vi "Finish.vi"   [LabVIEW 2015]
doc: "This VI is called just before exiting. It is expected to close I/O refnum, save collected data, etc."
uses:
  <vilib>/Rock Robotics/WPI/Utilities/WPI_GetSetVariantRefNum.vi
types:
  T1 = typedef "WPI_AccelerometerDevRef.ctl" = cluster{"DevStatus":errorcluster, "Scaling":T2, "Analog Channels":T3, "I2C Bus":T5, "SPI Bus":T6, "Accel Range":T7, "ADXL Axes":T8, "Handle":i32, "Device Address":u8, "Accel Type":enum16{"Analog", "ADXL345 I2C", "ADXL345 SPI", "Internal", "ADXL362 SPI"}}
  T2 = typedef "WPI_AccelerometerScaling.ctl" = cluster{"Gain (VoltsPerG)":dbl, "Center Voltage":dbl}
  T3 = typedef "WPI_AccelerometerAnalogChannels.ctl" = cluster{"X-Axis":T4, "Y-Axis":T4, "Z-Axis":T4}
  T4 = typedef "FPGA_AIChannel.ctl" = enum8{"AI 0", "AI 1", "AI 2", "AI 3", "AI MXP 0", "AI MXP 1", "AI MXP 2", "AI MXP 3", "Invalid"}
  T5 = typedef "i2c_bus.ctl" = enum16{"I2C On-Board", "I2C MXP", "Invalid"}
  T6 = typedef "spi_bus.ctl" = enum16{"SPI On-Board, CS0", "SPI On-Board, CS1", "SPI On-Board, CS2", "SPI On-Board, CS3", "SPI MXP", "Invalid"}
  T7 = typedef "ADXL345 Range.ctl" = u8
  T8 = typedef "WPI_AccelerometerADXL345 Axes.ctl" = cluster{"X-Axis":bool, "Y-Axis":bool, "Z-Axis":bool}
  T9 = typedef "WPI_DigitalInputDevRef.ctl" = cluster{"DevStatus":errorcluster, "DIO Channel":T10}
  T10 = typedef "FPGA_DIOChannel.ctl" = enum8{"DIO 0", "DIO 1", "DIO 2", "DIO 3", "DIO 4", "DIO 5", "DIO 6", "DIO 7", "DIO 8", "DIO 9", "DIO MXP 0", "DIO MXP 1", "DIO MXP 2", "DIO MXP 3", "DIO MXP 4", "DIO MXP 5", "DIO MXP 6", "DIO MXP 7", "DIO MXP 8", "DIO MXP 9", "DIO MXP 10", "DIO MXP 11", "DIO MXP 12", "DIO MXP 13", "DIO MXP 14", "DIO MXP 15", "Invalid"}
  T11 = typedef "WPI_GyroDevRef.ctl" = cluster{"DevStatus":errorcluster, "Analog Channel":T4, "Offset":dbl, "Gain (VoltsPerDegree/Second)":dbl, "Gyro Type":enum16{"Analog", "XRS450"}, "Handle":i32, "SPI Bus":T6, "Device Found":bool, "Sample Rate":dbl, "Calibrate On Open":bool}
  T12 = typedef "WPI_RelayDevRef.ctl" = cluster{"DevStatus":errorcluster, "Relay Channel":T13, "Relay Direction":T14}
  T13 = typedef "FPGA_DIORelayChannel.ctl" = enum8{"Relay 0", "Relay 1", "Relay 2", "Relay 3", "Invalid"}
  T14 = typedef "WPI_RelayDirection.ctl" = enum16{"Both directions", "Forward only", "Reverse only"}
  T15 = typedef "WPI_SolenoidDevRef.ctl" = cluster{"DevStatus":errorcluster, "Pneumatics Control Module":u8, "Forward Solenoid Channel":T16, "Reverse Solenoid Channel":T16}
  T16 = typedef "WPI_SolenoidChannel.ctl" = enum8{"Solenoid 0", "Solenoid 1", "Solenoid 2", "Solenoid 3", "Solenoid 4", "Solenoid 5", "Solenoid 6", "Solenoid 7", "Invalid"}
  T17 = typedef "WPI_EncoderDevRef.ctl" = cluster{"DevStatus":errorcluster, "EncoderIndex":T18, "CounterIndex":T19, "DistancePerCount":dbl, "Decoding Type":T20}
  T18 = typedef "FPGA_EncoderIdx.ctl" = enum8{"Enc 0", "Enc 1", "Enc 2", "Enc 3", "Enc 4", "Enc 5", "Enc 6", "Enc 7", "Invalid"}
  T19 = typedef "FPGA_CounterCtrSystemIndex.ctl" = enum8{"Ctr 0", "Ctr 1", "Ctr 2", "Ctr 3", "Ctr 4", "Ctr 5", "Ctr 6", "Ctr 7", "Invalid"}
  T20 = typedef "WPI_EncoderType.ctl" = enum16{"1x", "2x", "4x"}
  T21 = typedef "WPI_PotentiometerDevRef.ctl" = cluster{"DevStatus":errorcluster, "Analog Channel":T4, "Invert Output":bool}
  T22 = typedef "WPI_ServoDeviceRef.ctl" = cluster{"DeviceStatus":errorcluster, "PWM Channel":T23, "DeadBand":T24}
  T23 = typedef "FPGA_DIOPWMChannel.ctl" = enum8{"PWM 0", "PWM 1", "PWM 2", "PWM 3", "PWM 4", "PWM 5", "PWM 6", "PWM 7", "PWM 8", "PWM 9", "PWM MXP 0", "PWM MXP 1", "PWM MXP 2", "PWM MXP 3", "PWM MXP 4", "PWM MXP 5", "PWM MXP 6", "PWM MXP 7", "PWM MXP 8", "PWM MXP 9", "Invalid"}
  T24 = typedef "WPI_PWMDeadband.ctl" = cluster{"Name":string, "maxPositivePwm":i32, "minPositivePwm":i32, "centerPwm":i32, "maxNegativePwm":i32, "minNegativePwm":i32, "angularRange":u16}
  T25 = typedef "WPI_JoystickDevRef.ctl" = cluster{"Device":T26}
  T26 = typedef "WPI_JoystickDeviceEnum.ctl" = enum16{"USB 0", "USB 1", "USB 2", "USB 3", "USB 4", "USB 5"}
  T27 = typedef "WPI_MotorControlDeviceRef.ctl" = cluster{"DeviceStatus":errorcluster, "Type":T28, "PWM":cluster{"PWM Channel":T23, "DeadBand":T24}, "CAN":cluster{"Device Number":u8, "Control Mode":T29, "Semaphore":T30, "Max Vout":dbl, "TalonSRX Control Mode":T31}, "Invert":bool}
  T28 = typedef "WPI_MotorControlType.ctl" = enum16{"PWM", "CAN", "CANTalonSRX"}
  T29 = typedef "WPI_CANJaguar_ControlMode.ctl" = enum8{"Percent VBus", "Current", "Speed", "Position", "Voltage"}
  T30 = typedef "Semaphore RefNum" = refnum<k1>
  T31 = typedef "WPI_CANTalonSRX_APIControlMode.ctl" = enum8{"Percent VBus", "Speed", "Position", "Slave", "Unchanged / Invalid", "Voltage Compensation", "Current", "Motion Profile"}
  T32 = typedef "WPI_RobotDriveDevRef.ctl" = cluster{"DevStatus":errorcluster, "Motors[]":T27[], "Square Inputs":bool, "Max Output":dbl}
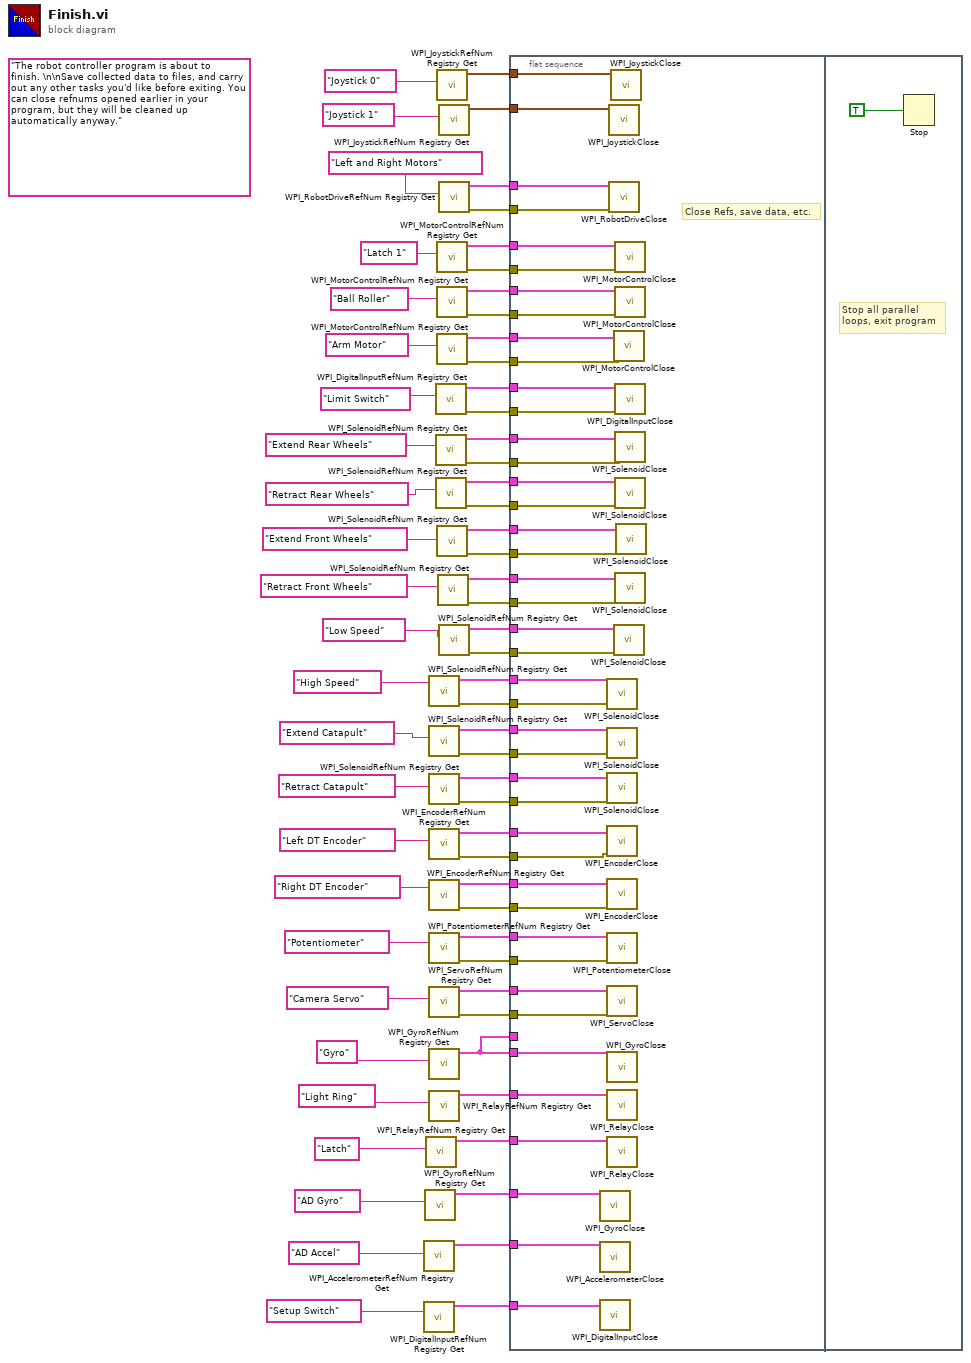
[diagram p0: block diagram]
diagram:
  (unwired) "The robot controller program is about to finish. \n\nSave collected data to files, and carry out any other tasks you'd like before exiting. You can close refnums opened earlier in your program, but they will be cleaned up automatically anyway."
  n1 = call <vilib>:"WPI_AccelerometerRefNum Registry Get.vi"("refnum name"="AD Accel") -> ("AccelerometerDevRef"=w5:T1)  [unwired: 9 in, 1 out]
  n2 = call <vilib>:"WPI_DigitalInputRefNum Registry Get.vi"("refnum name"="Setup Switch") -> ("DigitalInputDevRef"=w2:T9)  [unwired: 9 in, 1 out]
  n3 = call <vilib>:"WPI_GyroRefNum Registry Get.vi"("refnum name"="AD Gyro") -> ("GyroDevRef"=w6:T11)  [unwired: 9 in, 1 out]
  n4 = call <vilib>:"WPI_RelayRefNum Registry Get.vi"("refnum name"="Latch") -> ("RelayDevRef"=w8:T12)  [unwired: 9 in, 1 out]
  n5 = call <vilib>:"WPI_SolenoidRefNum Registry Get.vi"("refnum name"="High Speed") -> ("error out"=w29:errorcluster, "SolenoidDevRef"=w30:T15)  [unwired: 9 in]
  n6 = call <vilib>:"WPI_SolenoidRefNum Registry Get.vi"("refnum name"="Extend Catapult") -> ("error out"=w27:errorcluster, "SolenoidDevRef"=w28:T15)  [unwired: 9 in]
  n7 = call <vilib>:"WPI_SolenoidRefNum Registry Get.vi"("refnum name"="Retract Catapult") -> ("error out"=w25:errorcluster, "SolenoidDevRef"=w26:T15)  [unwired: 9 in]
  n8 = call <vilib>:"WPI_EncoderRefNum Registry Get.vi"("refnum name"="Left DT Encoder") -> ("error out"=w23:errorcluster, "EncoderDevRef"=w24:T17)  [unwired: 9 in]
  n9 = call <vilib>:"WPI_EncoderRefNum Registry Get.vi"("refnum name"="Right DT Encoder") -> ("error out"=w21:errorcluster, "EncoderDevRef"=w22:T17)  [unwired: 9 in]
  n10 = call <vilib>:"WPI_PotentiometerRefNum Registry Get.vi"("refnum name"="Potentiometer") -> ("error out"=w17:errorcluster, "PotDevRef"=w18:T21)  [unwired: 9 in]
  n11 = call <vilib>:"WPI_ServoRefNum Registry Get.vi"("refnum name"="Camera Servo") -> ("error out"=w14:errorcluster, "ServoDeviceRef"=w15:T22)  [unwired: 9 in]
  n12 = call <vilib>:"WPI_GyroRefNum Registry Get.vi"("refnum name"="Gyro") -> ("GyroDevRef"=w11:T11)  [unwired: 9 in, 1 out]
  n13 = call <vilib>:"WPI_RelayRefNum Registry Get.vi"("refnum name"="Light Ring") -> ("RelayDevRef"=w7:T12)  [unwired: 9 in, 1 out]
  n14 = call <vilib>:"WPI_DigitalInputRefNum Registry Get.vi"("refnum name"="Limit Switch") -> ("error out"=w49:errorcluster, "DigitalInputDevRef"=w57:T9)  [unwired: 9 in]
  n15 = call <vilib>:"WPI_SolenoidRefNum Registry Get.vi"("refnum name"="Extend Rear Wheels") -> ("error out"=w52:errorcluster, "SolenoidDevRef"=w53:T15)  [unwired: 9 in]
  n16 = call <vilib>:"WPI_SolenoidRefNum Registry Get.vi"("refnum name"="Retract Rear Wheels") -> ("error out"=w50:errorcluster, "SolenoidDevRef"=w51:T15)  [unwired: 9 in]
  n17 = call <vilib>:"WPI_JoystickRefNum Registry Get.vi"("refnum name"="Joystick 0") -> ("JoystickDevRef"=w58:T25)  [unwired: 1 in, 9 out]
  n18 = call <vilib>:"WPI_MotorControlRefNum Registry Get.vi"("refnum name"="Latch 1") -> ("error out"=w46:errorcluster, "MotorControlDevRef"=w63:T27)  [unwired: 9 in]
  n19 = call <vilib>:"WPI_MotorControlRefNum Registry Get.vi"("refnum name"="Ball Roller") -> ("error out"=w47:errorcluster, "MotorControlDevRef"=w61:T27)  [unwired: 9 in]
  n20 = call <vilib>:"WPI_MotorControlRefNum Registry Get.vi"("refnum name"="Arm Motor") -> ("error out"=w48:errorcluster, "MotorControlDevRef"=w55:T27)  [unwired: 9 in]
  n21 = call <vilib>:"WPI_SolenoidRefNum Registry Get.vi"("refnum name"="Extend Front Wheels") -> ("error out"=w43:errorcluster, "SolenoidDevRef"=w44:T15)  [unwired: 9 in]
  n22 = call <vilib>:"WPI_SolenoidRefNum Registry Get.vi"("refnum name"="Retract Front Wheels") -> ("error out"=w41:errorcluster, "SolenoidDevRef"=w42:T15)  [unwired: 9 in]
  n23 = call <vilib>:"WPI_JoystickRefNum Registry Get.vi"("refnum name"="Joystick 1") -> ("JoystickDevRef"=w64:T25)  [unwired: 1 in, 9 out]
  n24 = call <vilib>:"WPI_RobotDriveRefNum Registry Get.vi"("refnum name"="Left and Right Motors") -> ("error out"=w45:errorcluster, "RobotDriveDevRef"=w65:T32)  [unwired: 1 in, 8 out]
  n25 = call <vilib>:"WPI_SolenoidRefNum Registry Get.vi"("refnum name"="Low Speed") -> ("error out"=w35:errorcluster, "SolenoidDevRef"=w36:T15)  [unwired: 9 in]
  n26 = flat-sequence {
    tunnel: w65 -> [w109]
    tunnel: w64 -> [w108]
    tunnel: w63 -> [w107]
    tunnel: w61 -> [w106]
    tunnel: w58 -> [w105]
    tunnel: w57 -> [w104]
    tunnel: w55 -> [w103]
    tunnel: w53 -> [w102]
    tunnel: w52 -> [w101]
    tunnel: w51 -> [w100]
    tunnel: w50 -> [w99]
    tunnel: w49 -> [w98]
    tunnel: w48 -> [w97]
    tunnel: w47 -> [w96]
    tunnel: w46 -> [w95]
    tunnel: w45 -> [w94]
    tunnel: w44 -> [w93]
    tunnel: w43 -> [w92]
    tunnel: w42 -> [w91]
    tunnel: w41 -> [w90]
    tunnel: w36 -> [w89]
    tunnel: w35 -> [w88]
    tunnel: w30 -> [w87]
    tunnel: w29 -> [w86]
    tunnel: w28 -> [w85]
    tunnel: w27 -> [w84]
    tunnel: w26 -> [w83]
    tunnel: w25 -> [w82]
    tunnel: w24 -> [w81]
    tunnel: w23 -> [w80]
    tunnel: w22 -> [w79]
    tunnel: w21 -> [w78]
    tunnel: w18 -> [w77]
    tunnel: w17 -> [w76]
    tunnel: w15 -> [w75]
    tunnel: w14 -> [w74]
    tunnel: w11 -> [_]
    tunnel: w11 -> [w73]
    tunnel: w8 -> [w72]
    tunnel: w7 -> [w71]
    tunnel: w6 -> [w70]
    tunnel: w5 -> [w69]
    tunnel: w2 -> [w68]
    frame #0 {
      # "Close Refs, save data, etc."
      n27 = call <vilib>:"WPI_GyroClose.vi"("GyroDevRef"=w70) -> ()  [unwired: 10 in, 1 out]
      n28 = call <vilib>:"WPI_AccelerometerClose.vi"("AccelerometerDevRef"=w69) -> ()  [unwired: 10 in, 1 out]
      n29 = call <vilib>:"WPI_DigitalInputClose.vi"("DigitalInputDevRef"=w68) -> ()  [unwired: 10 in, 1 out]
      n30 = call <vilib>:"WPI_SolenoidClose.vi"("error in (no error)"=w86, "SolenoidDevRef"=w87) -> ()  [unwired: 9 in, 1 out]
      n31 = call <vilib>:"WPI_SolenoidClose.vi"("error in (no error)"=w84, "SolenoidDevRef"=w85) -> ()  [unwired: 9 in, 1 out]
      n32 = call <vilib>:"WPI_SolenoidClose.vi"("error in (no error)"=w82, "SolenoidDevRef"=w83) -> ()  [unwired: 9 in, 1 out]
      n33 = call <vilib>:"WPI_EncoderClose.vi"("error in (no error)"=w80, "EncoderDevRef"=w81) -> ()  [unwired: 9 in, 1 out]
      n34 = call <vilib>:"WPI_EncoderClose.vi"("error in (no error)"=w78, "EncoderDevRef"=w79) -> ()  [unwired: 9 in, 1 out]
      n35 = call <vilib>:"WPI_PotentiometerClose.vi"("error in"=w76, "PotDevRef"=w77) -> ()  [unwired: 9 in, 1 out]
      n36 = call <vilib>:"WPI_ServoClose.vi"("error in (no error)"=w74, "ServoDeviceRef"=w75) -> ()  [unwired: 9 in, 1 out]
      n37 = call <vilib>:"WPI_GyroClose.vi"("GyroDevRef"=w73) -> ()  [unwired: 10 in, 1 out]
      n38 = call <vilib>:"WPI_RelayClose.vi"("RelayDevRef"=w71) -> ()  [unwired: 10 in, 1 out]
      n39 = call <vilib>:"WPI_RelayClose.vi"("RelayDevRef"=w72) -> ()  [unwired: 10 in, 1 out]
      n40 = call <vilib>:"WPI_JoystickClose.vi"("JoystickDevRef"=w108) -> ()  [unwired: 11 out]
      n41 = call <vilib>:"WPI_RobotDriveClose.vi"("error in (no error)"=w94, "RobotDriveDevRef"=w109) -> ()  [unwired: 10 out]
      n42 = call <vilib>:"WPI_JoystickClose.vi"("JoystickDevRef"=w105) -> ()  [unwired: 11 out]
      n43 = call <vilib>:"WPI_MotorControlClose.vi"("error in (no error)"=w97, "MotorControlDevRef"=w103) -> ()  [unwired: 9 in, 1 out]
      n44 = call <vilib>:"WPI_SolenoidClose.vi"("error in (no error)"=w88, "SolenoidDevRef"=w89) -> ()  [unwired: 9 in, 1 out]
      n45 = call <vilib>:"WPI_MotorControlClose.vi"("error in (no error)"=w95, "MotorControlDevRef"=w107) -> ()  [unwired: 9 in, 1 out]
      n46 = call <vilib>:"WPI_MotorControlClose.vi"("error in (no error)"=w96, "MotorControlDevRef"=w106) -> ()  [unwired: 9 in, 1 out]
      n47 = call <vilib>:"WPI_DigitalInputClose.vi"("error in (no error)"=w98, "DigitalInputDevRef"=w104) -> ()  [unwired: 9 in, 1 out]
      n48 = call <vilib>:"WPI_SolenoidClose.vi"("error in (no error)"=w101, "SolenoidDevRef"=w102) -> ()  [unwired: 9 in, 1 out]
      n49 = call <vilib>:"WPI_SolenoidClose.vi"("error in (no error)"=w99, "SolenoidDevRef"=w100) -> ()  [unwired: 9 in, 1 out]
      n50 = call <vilib>:"WPI_SolenoidClose.vi"("error in (no error)"=w90, "SolenoidDevRef"=w91) -> ()  [unwired: 9 in, 1 out]
      n51 = call <vilib>:"WPI_SolenoidClose.vi"("error in (no error)"=w92, "SolenoidDevRef"=w93) -> ()  [unwired: 9 in, 1 out]
    }
    frame #1 {
      # "Stop all parallel\nloops, exit program"
      n52 = Stop(stop? (T)=TRUE ("Quit")) -> ()
    }
  }
